vi "Async Initialize.vi"(8 "error in (no error)":errorcluster, 10 "RT Configuration":T1={"Name"="", "Priority"=0, "XNET Settings"={"Database"="", "Cluster"="", "Port"="", "Baud rate [Bd]"=0, "Termination"=0, "CAN I/O Mode"=0, "FD Baud rate [Bd]"=500000, "Priority"=100, "Use Legacy"=FALSE, "FD ISO Mode"=0}, "FPGA Session"=0, "Outgoing CAN Session"="", "Outgoing Frame Count"=0, "Outgoing Frames"=[], "Incoming CAN Session"="", "Incoming Frame Count"=0, "Incoming Frames"=[], "Incoming Values"={"Signal Values"=[], "Signal Invalid Values"=[], "ProtCtr Sig Values"=[], "Timestamps"=[], "Time Differences"=[], "IDs"=[]}} {"Incoming Frames"."Protection Configurations"."CRC Channels"."Data Type" items=["Signed", "Unsigned", "IEEE Float"]; "XNET Settings"."FD ISO Mode" items=["ISO", "Non ISO", "ISO Legacy"]; "XNET Settings"."CAN I/O Mode" items=["CAN 2.0", "CAN FD", "CAN FD+BRS"]; "XNET Settings"."Termination" items=["Off", "On"]; "Outgoing Frames"."Protection Configurations"."CRC Channels"."Data Type" items=["Signed", "Unsigned", "IEEE Float"]}, 11 "Process in":refnum<class "Process.lvclass">) -> (0 "error out":errorcluster, 2 "Execute":bool, 3 "Variables":T11={"Process Ref"=refnum, "Comm Ref"=refnum, "Data Refs"={"ProtectionsAndCounters.Ref"=refnum, "Signals.Ref"=refnum, "Status.Ref"=refnum, "Overrides"=refnum, "IncomingSignals.Ref"=refnum, "CtrandProtctnVld.Ref"=refnum, "RcvTime.Ref"=refnum, "TimeDiff.Ref"=refnum, "IncomingProtCtr.Ref"=refnum}, "Settings"={"Name"="", "Priority"=0, "XNET Settings"={"Database"="", "Cluster"="", "Port"="", "Baud rate [Bd]"=0, "Termination"=0, "CAN I/O Mode"=0, "FD Baud rate [Bd]"=500000, "Priority"=100, "Use Legacy"=FALSE, "FD ISO Mode"=0}, "FPGA Session"=0, "Outgoing CAN Session"="", "Outgoing Frame Count"=0, "Outgoing Frames"=[], "Incoming CAN Session"="", "Incoming Frame Count"=0, "Incoming Frames"=[], "Incoming Values"={"Signal Values"=[], "Signal Invalid Values"=[], "ProtCtr Sig Values"=[], "Timestamps"=[], "Time Differences"=[], "IDs"=[]}}, "Stream Refs"={"Addon"="", "Port"="", "Filter Ref"=refnum, "Default Filter"={"ID Filters"=[], "Direction Filter"=enum."Tx/Rx", "Type Filter"=enum."All"}, "Port Settings"={"Mode"=0, "Baud Rate"=0, "Termination"=0, "FD ISO Mode"=0, "FD Baud Rate"=0}}} {"Stream Refs"."Port Settings"."FD ISO Mode" items=["ISO", "Non ISO", "ISO Legacy"]; "Stream Refs"."Port Settings"."Termination" items=["Off", "On"]; "Stream Refs"."Port Settings"."Mode" items=["CAN 2.0", "CAN FD", "CAN FD+BRS"]; "Settings"."XNET Settings"."FD ISO Mode" items=["ISO", "Non ISO", "ISO Legacy"]; "Settings"."XNET Settings"."CAN I/O Mode" items=["CAN 2.0", "CAN FD", "CAN FD+BRS"]; "Settings"."XNET Settings"."Termination" items=["Off", "On"]})   [LabVIEW 2023, in "Protection and Counter Addon Engine.lvlib"]
uses:
  Protection and Counter Addon Engine.lvlib
  Types/RT Async Engine Variables.ctl
  <vilib>/NI/NIVS Inline Async API/_VS Inline Async API/Process/Process.lvclass
  <vilib>/NI/NI VeriStand Addon Network Comm/Engine/VeriStand Comm.lvclass
  Types/RT Data References.ctl
  <vilib>/NI/NIVS Inline Async API/_Data Access Engine/Data Access Engine/Types/Write.DVR.ctl
  <vilib>/NI/NIVS Inline Async API/_Data Access Engine/Access Type Classes/Write/Write.lvclass
  <vilib>/NI/NIVS Inline Async API/_Data Access Engine/Data Access Engine/Types/Read.DVR.ctl
  <vilib>/NI/NIVS Inline Async API/_Data Access Engine/Access Type Classes/Read/Read.lvclass
  Types/RT Async Engine Settings.ctl
  Addon Shared/Types/XNET Settings.ctl
  SubModules/Frame-Protection-Support/Source/Engine/Types/RT Frame Settings.ctl
  SubModules/Frame-Protection-Support/Source/Shared/Types/Exported Frame Type.ctl
  SubModules/Frame-Protection-Support/Source/Engine/Types/RT Protection Configuration.ctl
  SubModules/Frame-Protection-Support/Source/Shared/Types/Protection Type.ctl
  SubModules/Frame-Protection-Support/Source/Shared/Types/XNET Signal Configuration.ctl
  SubModules/Frame-Protection-Support/Source/Shared/Types/Exported Counter Settings.ctl
  SubModules/Frame-Protection-Support/Source/Shared/Types/Exported Event Trigger Type.ctl
  SubModules/Frame-Protection-Support/Source/Engine/Types/RT Frame Incoming Values.ctl
  SubModules/CAN-Streaming-Support/Source/Addon/Addon Engine/Types/Engine Stream Refs.ctl
  SubModules/CAN-Streaming-Support/Source/Addon/Addon Shared/Types/Direction Filter.ctl
  SubModules/CAN-Streaming-Support/Source/Addon/Addon Shared/Types/Type Filter.ctl
  SubModules/CAN-Streaming-Support/Source/Addon/Addon Shared/Types/Filter Parameters.ctl
  SubModules/CAN-Streaming-Support/Source/Addon/Addon Engine/Types/Engine Stream Port Settings.ctl
  <vilib>/NI/NI VeriStand Addon Network Comm/Engine/VeriStand Comm.lvclass/VeriStand Comm.ctl
  <vilib>/NI/NIVS Inline Async API/_VS Inline Async API/Process/Process.lvclass/Process.ctl
  <vilib>/NI/NIVS Inline Async API/_VS Inline Async API/Process/Data Member Access/Read Data Access.vi
  <vilib>/NI/NIVS Inline Async API/_VS Inline Async API/Error Handling Process/SubVIs/Error.ConvertArray.vi
  Addon Shared/SubVIs/GUID Lookup.vi
  <vilib>/Utility/SystemLogging/Write to System Log.vi
  <vilib>/NI/AMC/Create Message Queue.vi
  <vilib>/NI/STM/Connection Manager/TCP/Advanced/TCP Initialize Connection Manager (By Reference).vi
  <vilib>/NI/NIVS Inline Async API/_Data Access Engine/Data Access Engine/Methods/Read.Lookup.vi
  <vilib>/NI/NIVS Inline Async API/_Data Access Engine/Data Access Engine/Methods/Write.Lookup.vi
  <vilib>/NI/NIVS Inline Async API/_Data Access Engine/Data Access Engine/Data Access Engine.lvclass
  Addon Shared/Protection and Counter Addon Shared.lvlib
  SubModules/Frame-Protection-Support/Source/Shared/Protection and Counter Support Shared.lvlib
  SubModules/Frame-Protection-Support/Source/Engine/Protection and Counter Support Engine.lvlib
  SubModules/CAN-Streaming-Support/Source/Addon/Addon Shared/CAN Stream Support Shared.lvlib
  SubModules/CAN-Streaming-Support/Source/Addon/Addon Engine/CAN Stream Support Engine.lvlib
  <resource>/objmgr/xnet.rc
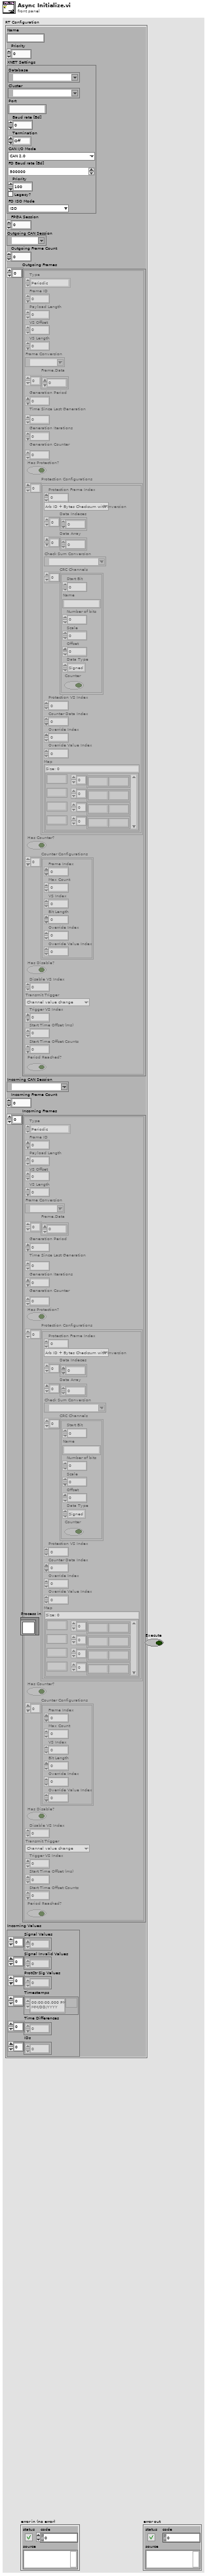
[diagram p1: front panel]
types:
  T1 = typedef "Protection and Counter Addon Engine.lvlib/RT Async Engine Settings.ctl" = cluster{"Name":string, "Priority":i32, "XNET Settings":T2, "FPGA Session":u32, "Outgoing CAN Session":refnum<k21>, "Outgoing Frame Count":i32, "Outgoing Frames":T3[], "Incoming CAN Session":refnum<k21>, "Incoming Frame Count":i32, "Incoming Frames":T3[], "Incoming Values":T10}
  T2 = typedef "Protection and Counter Addon Shared.lvlib/XNET Settings.ctl" = cluster{"Database":refnum<k21>, "Cluster":refnum<k21>, "Port":string, "Baud rate [Bd]":u64, "Termination":u32, "CAN I/O Mode":u32, "FD Baud rate [Bd]":u64, "Priority":i32, "Use Legacy":bool, "FD ISO Mode":u32}
  T3 = typedef "Protection and Counter Support Engine.lvlib/RT Frame Settings.ctl" = cluster{"Type":T4, "Frame ID":u32, "Payload Length":u32, "VS Offset":i32, "VS Length":i32, "Frame Conversion":refnum<k21>, "Frame.Data":dbl[], "Generation Period":u32, "Time Since Last Generation":u32, "Generation Iterations":u32, "Generation Counter":u32, "Has Protection?":bool, "Protection Configurations":T5[], "Has Counter?":bool, "Counter Configurations":T8[], "Has Disable?":bool, "Disable VS Index":i32, "Transmit Trigger":T9, "Trigger VS Index":i32, "Start Time Offset (ms)":u32, "Start Time Offset Counts":u32, "Period Reached?":bool}
  T4 = typedef "Protection and Counter Support Shared.lvlib/Exported Frame Type.ctl" = enum16{"Periodic", "Event", "Periodic/Event"}
  T5 = typedef "Protection and Counter Support Engine.lvlib/RT Protection Configuration.ctl" = cluster{"Protection Frame Index":i32, "Protection Type":T6, "Data Indeces":i32[], "Data Array":dbl[], "Check Sum Conversion":refnum<k21>, "CRC Channels":T7[], "Protection VS Index":i32, "Counter Data Index":i32, "Override Index":i32, "Override Value Index":i32, "Map":map{i32, u8[]}}
  T6 = typedef "Protection and Counter Support Shared.lvlib/Protection Type.ctl" = enum16{"Arb ID + Bytes Checksum with Inversion", "Arb ID + Bytes CRC with Inversion", "Reversed Raw Signal Checksum with Inversion", "Concatenated Two's Compliment", "LP_CRC8", "LP_Checksum", "LP_CRC8_MRS"}
  T7 = typedef "Protection and Counter Support Shared.lvlib/XNET Signal Configuration.ctl" = cluster{"Start Bit":i32, "Name":string, "Number of bits":i32, "Scale":dbl, "Offset":dbl, "Data Type":u32, "Counter":bool}
  T8 = typedef "Protection and Counter Support Shared.lvlib/Exported Counter Settings.ctl" = cluster{"Frame Index":i32, "Max Count":dbl, "VS Index":i32, "Bit Length":i64, "Override Index":i32, "Override Value Index":i32}
  T9 = typedef "Protection and Counter Support Shared.lvlib/Exported Event Trigger Type.ctl" = enum16{"Channel value change", "Trigger channel (not zero)", "Channel value change or trigger channel (not zero)", "Trigger channel (any value change)", "Channel value change or trigger channel (any value change)"}
  T10 = typedef "Protection and Counter Support Engine.lvlib/RT Frame Incoming Values.ctl" = cluster{"Signal Values":dbl[], "Signal Invalid Values":dbl[], "ProtCtr Sig Values":dbl[], "Timestamps":timestamp[], "Time Differences":dbl[], "IDs":u32[]}
  T11 = typedef "Protection and Counter Addon Engine.lvlib/RT Async Engine Variables.ctl" = cluster{"Process Ref":refnum<class "Process.lvclass">, "Comm Ref":refnum<class "VeriStand Comm.lvclass">, "Data Refs":T12, "Settings":T1, "Stream Refs":T15}
  T12 = typedef "Protection and Counter Addon Engine.lvlib/RT Data References.ctl" = cluster{"ProtectionsAndCounters.Ref":T13, "Signals.Ref":T14, "Status.Ref":T13, "Overrides":T14, "IncomingSignals.Ref":T13, "CtrandProtctnVld.Ref":T13, "RcvTime.Ref":T13, "TimeDiff.Ref":T13, "IncomingProtCtr.Ref":T13}
  T13 = typedef "Data Access Engine.lvlib/Data Access Engine.lvclass/Write.DVR.ctl" = refnum<data-value>
  T14 = typedef "Data Access Engine.lvlib/Data Access Engine.lvclass/Read.DVR.ctl" = refnum<data-value>
  T15 = typedef "CAN Stream Support Engine.lvlib/Engine Stream Refs.ctl" = cluster{"Addon":string, "Port":refnum<k21>, "Filter Ref":refnum<data-value>, "Default Filter":T16, "Port Settings":T19}
  T16 = typedef "CAN Stream Support Shared.lvlib/Filter Parameters.ctl" = cluster{"ID Filters":u32[], "Direction Filter":T17, "Type Filter":T18}
  T17 = typedef "CAN Stream Support Shared.lvlib/Direction Filter.ctl" = enum16{"Tx/Rx", "Rx", "Tx"}
  T18 = typedef "CAN Stream Support Shared.lvlib/Type Filter.ctl" = enum16{"All", "CAN Data", "CAN Remote", "CAN Bus Error", "CAN 2.0 Data", "CAN FD Data", "CAN FD+BRS Data", "J1939 Data", "Delay", "Log Trigger", "Start Trigger"}
  T19 = typedef "CAN Stream Support Engine.lvlib/Engine Stream Port Settings.ctl" = cluster{"Mode":u32, "Baud Rate":u64, "Termination":u32, "FD ISO Mode":u32, "FD Baud Rate":u64}
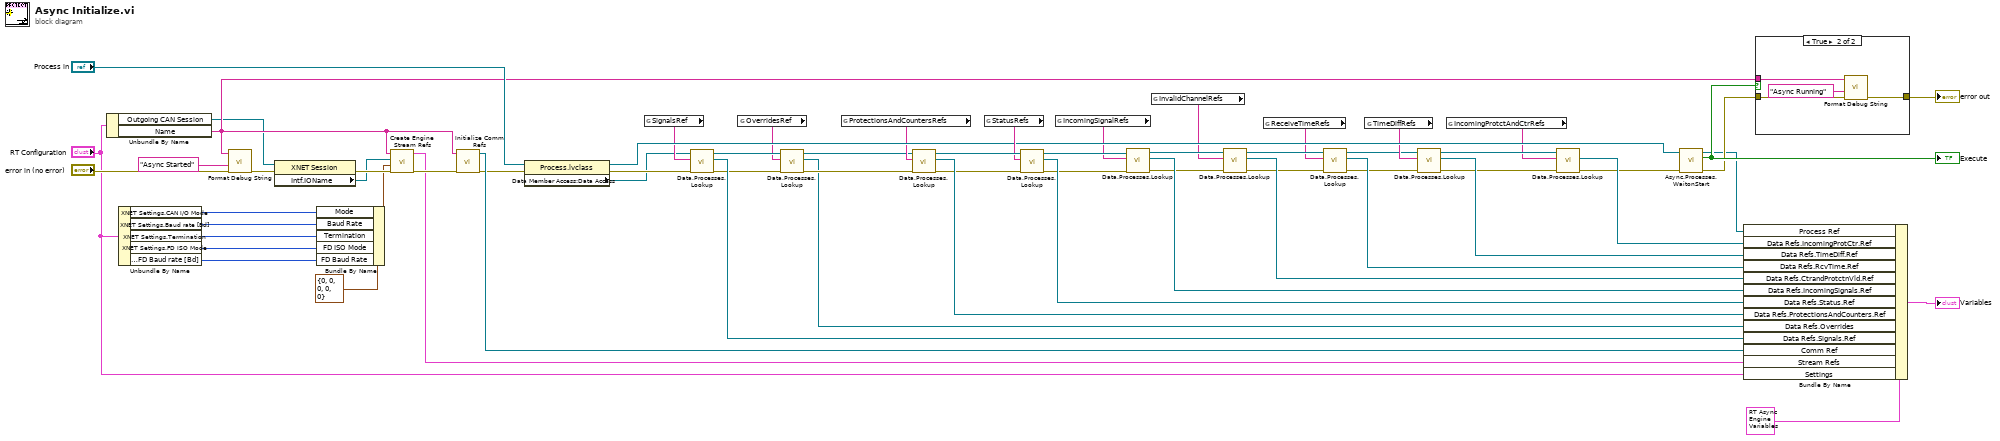
[diagram p0: block diagram]
diagram:
  n1 = Unbundle By Name("RT Configuration") -> ("Outgoing CAN Session"=w39:refnum<k21>, "Name"=w40:string)
  n2 = Unbundle By Name("RT Configuration") -> ("XNET Settings.CAN I/O Mode"=w27:u32, "XNET Settings.Baud rate [Bd]"=w24:u64, "XNET Settings.Termination"=w25:u32, "XNET Settings.FD ISO Mode"=w23:u32, "XNET Settings.FD Baud rate [Bd]"=w26:u64)
  n3 = call "Format Debug String.vi"("error in (no error)"="error in (no error)", "State"="Async Started", "Name"=w40) -> ("error out"=w42:errorcluster)  [unwired: 8 in]
  n4 = property class="XNET Session"(reference=w39, error in=w42) -> (error out=w41:errorcluster, "Intf.IOName"=w38:refnum<k21>)  [unwired: 1 out]
  n5 = Bundle By Name(cluster=T19 {"Mode"=0, "Baud Rate"=0, "Termination"=0, "FD ISO Mode"=0, "FD Baud Rate"=0} ("Port Settings"), "Mode"=w27, "Baud Rate"=w24, "Termination"=w25, "FD ISO Mode"=w23, "FD Baud Rate"=w26) -> (w28:T19)
  n6 = call "Create Engine Stream Refs.vi"("error in (no error)"=w41, "Port Settings"=w28, "Port"=w38, "Addon"=w40) -> ("error out"=w43:errorcluster, "Refs"=w37:T15)  [unwired: 6 in]
  n7 = call <vilib>:"Initialize Comm Refs.vi"("error in (no error)"=w43, "Name"=w40) -> ("error out"=w58:errorcluster, "Comm.lvclass"=w64:refnum<class "VeriStand Comm.lvclass">)  [unwired: 8 in]
  n8 = property class="Process.lvclass"(reference="Process in", error in=w58) -> (reference out=w49:refnum<class "Process.lvclass">, error out=w46:errorcluster, "Data Member Access:Data Access"=w45:refnum<class "Data Access Engine.lvclass">)
  n9 = global read "GUID Lookup.vi" "SignalsRef"() -> (w47:string)
  n10 = call-poly <vilib>:"Data.Processes.Lookup.vi"("error in (no error)"=w46, "Name"=w47, "Data Access API in"=w45) -> ("error out"=w36:errorcluster, "Ref"=w63:T14, "Data Access API out"=w34:refnum<class "Data Access Engine.lvclass">)  [unwired: 5 in, 1 out]
  n11 = global read "GUID Lookup.vi" "OverridesRef"() -> (w32:string)
  n12 = call-poly <vilib>:"Data.Processes.Lookup.vi"("error in (no error)"=w36, "Name"=w32, "Data Access API in"=w34) -> ("error out"=w35:errorcluster, "Ref"=w31:T14, "Data Access API out"=w33:refnum<class "Data Access Engine.lvclass">)  [unwired: 5 in, 1 out]
  n13 = global read "GUID Lookup.vi" "ProtectionsAndCountersRefs"() -> (w48:string)
  n14 = call-poly <vilib>:"Data.Processes.Lookup.vi"("error in (no error)"=w35, "Name"=w48, "Data Access API in"=w33) -> ("error out"=w52:errorcluster, "Ref"=w62:T13, "Data Access API out"=w51:refnum<class "Data Access Engine.lvclass">)  [unwired: 5 in, 1 out]
  n15 = global read "GUID Lookup.vi" "StatusRefs"() -> (w50:string)
  n16 = call-poly <vilib>:"Data.Processes.Lookup.vi"("error in (no error)"=w52, "Name"=w50, "Data Access API in"=w51) -> ("error out"=w6:errorcluster, "Ref"=w61:T13, "Data Access API out"=w22:refnum<class "Data Access Engine.lvclass">)  [unwired: 5 in, 1 out]
  n17 = global read "GUID Lookup.vi" "IncomingSignalRefs"() -> (w19:string)
  n18 = call-poly <vilib>:"Data.Processes.Lookup.vi"("error in (no error)"=w6, "Name"=w19, "Data Access API in"=w22) -> ("error out"=w5:errorcluster, "Ref"=w13:T13, "Data Access API out"=w21:refnum<class "Data Access Engine.lvclass">)  [unwired: 5 in, 1 out]
  n19 = global read "GUID Lookup.vi" "InvalidChannelRefs"() -> (w18:string)
  n20 = call-poly <vilib>:"Data.Processes.Lookup.vi"("error in (no error)"=w5, "Name"=w18, "Data Access API in"=w21) -> ("error out"=w4:errorcluster, "Ref"=w15:T13, "Data Access API out"=w20:refnum<class "Data Access Engine.lvclass">)  [unwired: 5 in, 1 out]
  n21 = global read "GUID Lookup.vi" "ReceiveTimeRefs"() -> (w17:string)
  n22 = call-poly <vilib>:"Data.Processes.Lookup.vi"("error in (no error)"=w4, "Name"=w17, "Data Access API in"=w20) -> ("error out"=w3:errorcluster, "Ref"=w14:T13, "Data Access API out"=w11:refnum<class "Data Access Engine.lvclass">)  [unwired: 5 in, 1 out]
  n23 = global read "GUID Lookup.vi" "TimeDiffRefs"() -> (w12:string)
  n24 = call-poly <vilib>:"Data.Processes.Lookup.vi"("error in (no error)"=w3, "Name"=w12, "Data Access API in"=w11) -> ("error out"=w2:errorcluster, "Ref"=w10:T13, "Data Access API out"=w9:refnum<class "Data Access Engine.lvclass">)  [unwired: 5 in, 1 out]
  n25 = global read "GUID Lookup.vi" "IncomingProtctAndCtrRefs"() -> (w8:string)
  n26 = call-poly <vilib>:"Data.Processes.Lookup.vi"("error in (no error)"=w2, "Name"=w8, "Data Access API in"=w9) -> ("error out"=w1:errorcluster, "Ref"=w7:T13)  [unwired: 5 in, 2 out]
  n27 = call <vilib>:"Async.Processes.WaitonStart.vi"("error in (no error)"=w1, "Process"=w49) -> ("error out"=w55:errorcluster, "Execute"=w57:bool, "Process out"=w16:refnum<class "Process.lvclass">)  [unwired: 7 in]
  "Execute" <- w57
  n28 = Bundle By Name(cluster=T11 {"Process Ref"=refnum, "Comm Ref"=refnum, "Data Refs"={"ProtectionsAndCounters.Ref"=refnum, "Signals.Ref"=refnum, "Status.Ref"=refnum, "Overrides"=refnum, "IncomingSignals.Ref"=refnum, "CtrandProtctnVld.Ref"=refnum, "RcvTime.Ref"=refnum, "TimeDiff.Ref"=refnum, "IncomingProtCtr.Ref"=refnum}, "Settings"={"Name"="", "Priority"=0, "XNET Settings"={"Database"="", "Cluster"="", "Port"="", "Baud rate [Bd]"=0, "Termination"=0, "CAN I/O Mode"=0, "FD Baud rate [Bd]"=500000, "Priority"=100, "Use Legacy"=FALSE, "FD ISO Mode"=0}, "FPGA Session"=0, "Outgoing CAN Session"="", "Outgoing Frame Count"=0, "Outgoing Frames"=[], "Incoming CAN Session"="", "Incoming Frame Count"=0, "Incoming Frames"=[], "Incoming Values"={"Signal Values"=[], "Signal Invalid Values"=[], "ProtCtr Sig Values"=[], "Timestamps"=[], "Time Differences"=[], "IDs"=[]}}, "Stream Refs"={"Addon"="", "Port"="", "Filter Ref"=refnum, "Default Filter"={"ID Filters"=[], "Direction Filter"=enum."Tx/Rx", "Type Filter"=enum."All"}, "Port Settings"={"Mode"=0, "Baud Rate"=0, "Termination"=0, "FD ISO Mode"=0, "FD Baud Rate"=0}}}, "Process Ref"=w16, "Data Refs.IncomingProtCtr.Ref"=w7, "Data Refs.TimeDiff.Ref"=w10, "Data Refs.RcvTime.Ref"=w14, "Data Refs.CtrandProtctnVld.Ref"=w15, "Data Refs.IncomingSignals.Ref"=w13, "Data Refs.Status.Ref"=w61, "Data Refs.ProtectionsAndCounters.Ref"=w62, "Data Refs.Overrides"=w31, "Data Refs.Signals.Ref"=w63, "Comm Ref"=w64, "Stream Refs"=w37, "Settings"="RT Configuration") -> (→"Variables":T11)
  n29 = case shown="True" w57 {
    tunnel: w55 -> [w65 w68]
    tunnel: [w65 w67] -> w56
    tunnel: w40 -> [_ w66]
    frame False {
    }
    frame True {
      n30 = call "Format Debug String.vi"("error in (no error)"=w68, "State"="Async Running", "Name"=w66) -> ("error out"=w67:errorcluster)  [unwired: 8 in]
    }
  }
  "error out" <- w56
